vi "Close.vi"(8 "error in (no error)":errorcluster, 11 "SLL Subpanel Manager in":refnum<class "SLL Subpanel Manager.lvclass">) -> (0 "error out":errorcluster)   [LabVIEW 2016, in "SLL Subpanel Manager.lvclass"]
uses:
  SLL Subpanel Manager.lvclass
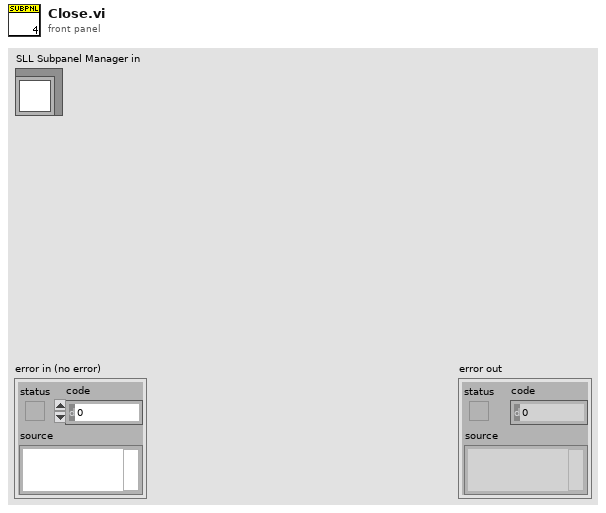
[diagram p1: front panel]
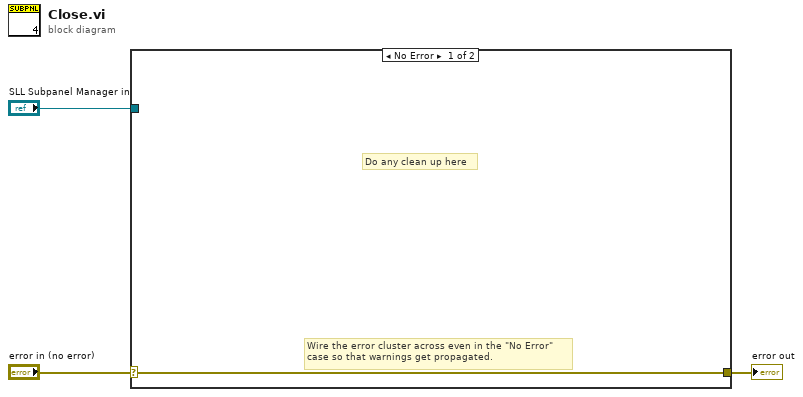
[diagram p0: block diagram]
diagram:
  n1 = case shown="No Error" "error in (no error)" {
    selector: "error in (no error)" -> [w4 w5]
    tunnel: [w4 w5] -> w2
    tunnel: "SLL Subpanel Manager in" -> [_ _]
    frame No Error {
      # "Do any clean up here"
      # "Wire the error cluster across even in the \"No Error\"\ncase so that warnings get propagated."
    }
    frame Error {
    }
  }
  "error out" <- w2
